vi "Handle.vi"(7 "Queue Actor in":refnum<class "Queue Actor.lvclass">, 11 "Nominal Queue State in":refnum<class "Nominal Queue State.lvclass">) -> (2 "Destroy?":bool, 5 "Queue Actor out":refnum<class "Queue Actor.lvclass">)   [LabVIEW 2021, in "jettl.lvlib" / "Nominal Queue State.lvclass"]
uses:
  Nominal Queue State.lvclass
  Actor/Queue Actor/Queue Actor.lvclass
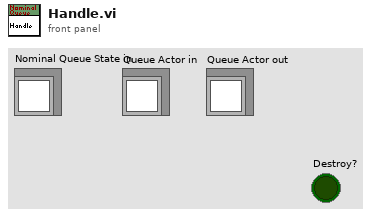
[diagram p1: front panel]
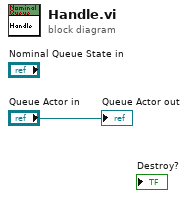
[diagram p0: block diagram]
diagram:
  "Queue Actor out" <- "Queue Actor in"
